vi "imgwindow.vi"(0 "String":string, 1 "File Path":path, 2 "sync":bool, 3 "inf array":dbl[][](array[numeric]), 4 "Image 2":T1, 5 "error in (no error)":errorcluster, 6 "last difrence":i32) -> (14 "This VI":refnum<vi>, 18 "error out":errorcluster)   [LabVIEW 2019]
uses:
  <vilib>/vision/Image Controls.llb/IMAQ Image.ctl
panel:
  out "ALARM":bool
  out "SYNC":bool
  out "Frm false":bool
  out "Pallet Analyzed":T1(plugin-control)
  out "SWL":bool
  out "SWR":bool
  out "PLT num":string="178"
  out "curv def":bool
  out "GB def":bool
  out "CURV":string
  out "GRBR":string="2"
  out "DEF type":string="1"
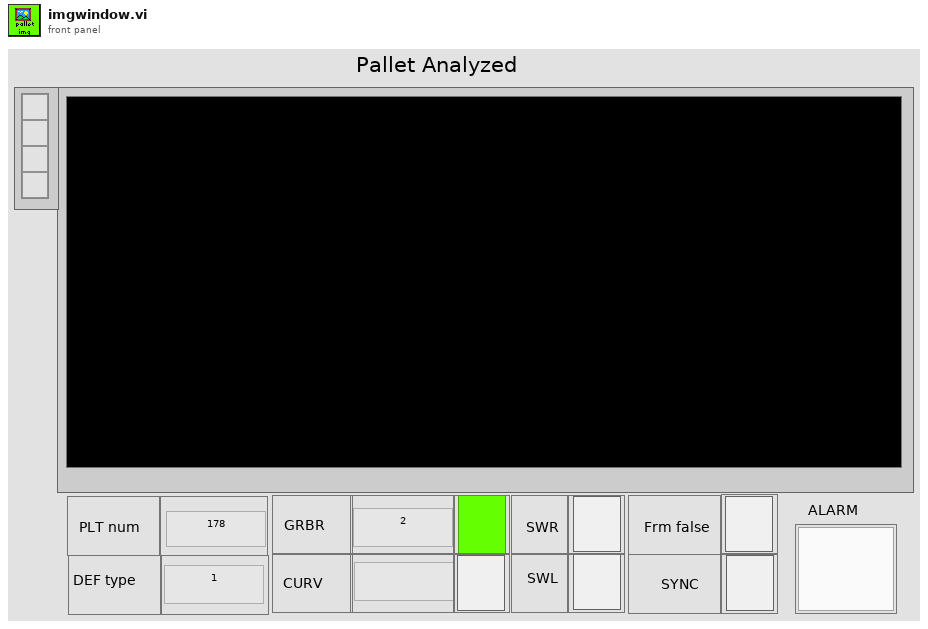
[diagram p1: front panel]
types:
  T1 = typedef "IMAQ Image.ctl" = refnum<image>
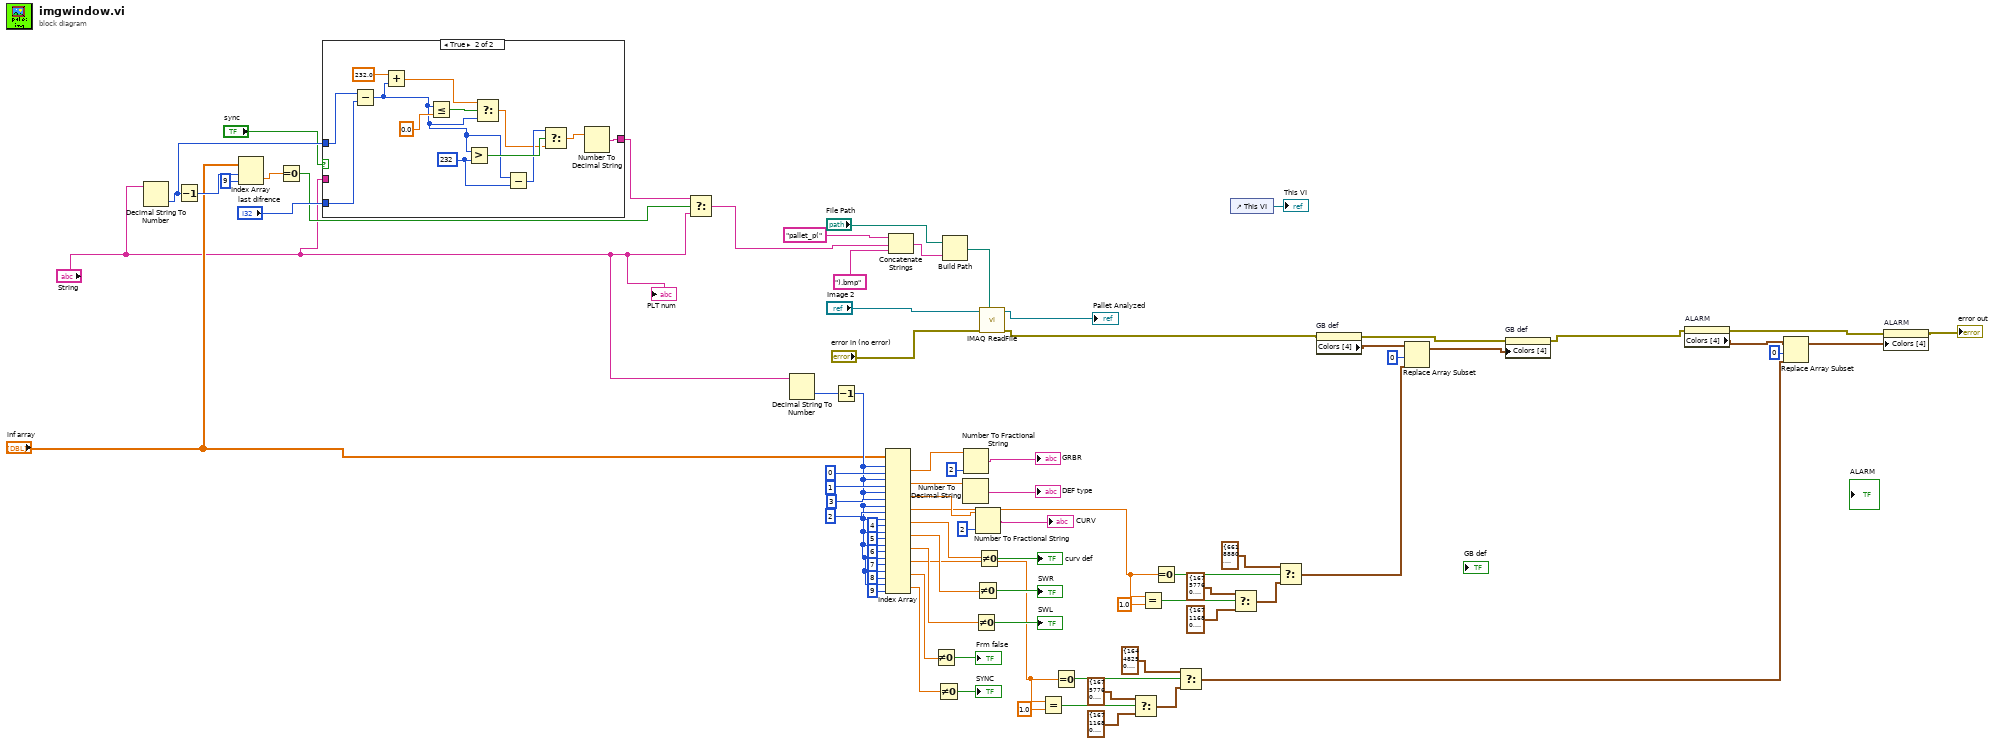
[diagram p0: block diagram]
diagram:
  n1 = Decimal String To Number(string="String") -> (number=w7:i32)  [unwired: 2 in, 1 out]
  n2 = Decrement(x=w7) -> (x-1=w10:i32)
  n3 = Index Array(array="inf array", index (row)=w10, index (col)=9 ("disabled index (col)")) -> (element=w8:dbl)
  n4 = Equal To 0?(x=w8) -> (x = 0?=w4:bool)
  n5 = case shown="True" "sync" {
    tunnel: w7 -> [_ w88]
    tunnel: [w80 w89] -> w3
    tunnel: "String" -> [w80 _]
    tunnel: "last difrence" -> [_ w87]
    frame False {
    }
    frame True {
      w82 = 232 ("y")
      n6 = Subtract(x=w88, y=w87) -> (x-y=w81:i32)
      n7 = Add(x=232.0, y=w81) -> (x+y=w90:dbl)
      n8 = Less Or Equal?(x=w81, y=0.0) -> (x <= y?=w93:bool)
      n9 = Greater?(x=w81, y=w82) -> (0:w86:bool)
      n10 = Select(t=w90, s=w93, f=w81) -> (s? t:f=w84:dbl)
      n11 = Subtract(x=w81, y=w82) -> (x-y=w85:i32)
      n12 = Select(t=w85, s=w86, f=w84) -> (s? t:f=w83:dbl)
      n13 = Number To Decimal String(number=w83) -> (decimal integer string=w89:string)  [unwired: 1 in]
    }
  }
  n14 = Select(t=w3, s=w4, f="String") -> (s? t:f=w1:string)
  n15 = Decimal String To Number(string="String") -> (number=w68:i32)  [unwired: 2 in, 1 out]
  n16 = Decrement(x=w68) -> (x-1=w18:i32)
  n17 = Index Array(array="inf array", index (row) #1=w18, index (col) #1=0 ("disabled index (col)"), index (row) #2=w18, index (col) #2=1 ("disabled index (col)"), index (row) #3=w18, index (col) #3=3 ("disabled index (col)"), index (row) #4=w18, index (col) #4=2 ("disabled index (col)"), index (row) #5=w18, index (col) #5=4 ("disabled index (col)"), index (row) #6=w18, index (col) #6=5 ("disabled index (col)"), index (row) #7=w18, index (col) #7=6 ("disabled index (col)"), index (row) #8=w18, index (col) #8=7 ("disabled index (col)"), index (row) #9=w18, index (col) #9=8 ("disabled index (col)"), index (row) #10=w18, index (col) #10=9 ("disabled index (col)")) -> (element #1=w64:dbl, element #2=w72:dbl, element #3=w61:dbl, element #4=w56:dbl, element #5=w46:dbl, element #6=w44:dbl, element #7=w40:dbl, element #8=w30:dbl, element #9=w12:dbl, element #10=w14:dbl)
  n18 = Concatenate Strings("pallet_p(" ("string"), w1, ").bmp" ("string")) -> (w67:string)
  n19 = Not Equal To 0?(x=w12) -> (x != 0?=→"Frm false":bool)
  n20 = Not Equal To 0?(x=w14) -> (x != 0?=→"SYNC":bool)
  n21 = Build Path(base path="File Path", name or relative path=w67) -> (appended path=w75:path)
  n22 = Number To Decimal String(number=w72) -> (decimal integer string=→"DEF type":string)  [unwired: 1 in]
  n23 = Number To Fractional String(number=w64, precision (6)=i16 2) -> (F-format string=→"GRBR":string)  [unwired: 2 in]
  n24 = Not Equal To 0?(x=w40) -> (x != 0?=→"SWL":bool)
  n25 = Number To Fractional String(number=w61, precision (6)=i16 2) -> (F-format string=→"CURV":string)  [unwired: 2 in]
  n26 = Not Equal To 0?(x=w44) -> (x != 0?=→"SWR":bool)
  n27 = Not Equal To 0?(x=w46) -> (x != 0?=→"curv def":bool)
  n28 = call "IMAQ ReadFile"("File Path"=w75, "error in (no error)"="error in (no error)", "Image"="Image 2") -> ("error out"=w23:errorcluster, "Image Out"=→"Pallet Analyzed":T1)  [unwired: 4 in, 3 out]
  n29 = Equal?(x=w30, y=1.0) -> (x = y?=w33:bool)
  n30 = Equal To 0?(x=w30) -> (x = 0?=w31:bool)
  n31 = Select(t=cluster{u32, u32} {16757760, 16763714} ("new element/subarray"), s=w33, f=cluster{u32, u32} {16711680, 16711680} ("new element/subarray")) -> (s? t:f=w37:cluster{u32, u32})
  n32 = Equal?(x=w56, y=1.0) -> (x = y?=w54:bool)
  n33 = Equal To 0?(x=w56) -> (x = 0?=w57:bool)
  n34 = Select(t=cluster{u32, u32} {16448250, 16448250} ("new element/subarray"), s=w31, f=w37) -> (s? t:f=w27:cluster{u32, u32})
  n35 = control-ref of="This VI"() -> (→"This VI":refnum<vi>)
  n36 = Select(t=cluster{u32, u32} {16757760, 16763714} ("new element/subarray"), s=w54, f=cluster{u32, u32} {16711680, 16711680} ("new element/subarray")) -> (s? t:f=w50:cluster{u32, u32})
  n37 = Select(t=cluster{u32, u32} {6618880, 6618880} ("new element/subarray"), s=w57, f=w50) -> (s? t:f=w48:cluster{u32, u32})
  n38 = property on="GB def" class="Bool"(error in=w23) -> (error out=w20:errorcluster, "Colors [4]"=w22:cluster{u32, u32}[])  [unwired: 1 in, 1 out]
  n39 = Replace Array Subset(array=w22, new element=w48, index=0) -> (w21:cluster{u32, u32}[])
  n40 = property on="GB def" class="Bool"(error in=w20, "Colors [4]"=w21) -> (error out=w19:errorcluster)  [unwired: 1 in, 1 out]
  n41 = property on="ALARM" class="Bool (strict)"(error in=w19) -> (error out=w25:errorcluster, "Colors [4]"=w28:cluster{u32, u32}[])  [unwired: 1 in, 1 out]
  n42 = Replace Array Subset(array=w28, new element=w27, index=0) -> (w26:cluster{u32, u32}[])
  n43 = property on="ALARM" class="Bool (strict)"(error in=w25, "Colors [4]"=w26) -> (error out=→"error out":errorcluster)  [unwired: 1 in, 1 out]
  "PLT num" <- "String"
